vi "SetAdapTorrLocal_v0.vi"(2 "Debug Mode":bool, 3 "Elapsed Time (s)":dbl, 4 "State":enum16{"Edit", "Start", "Run", "End", "Idle"}(ring), 5 "Argument List In":string[](array[string])) -> (0 "Status Out":string, 1 "Argument List Out":string[](array[string]))   [LabVIEW 2011]
panel:
  in  "error in (no error)":errorcluster
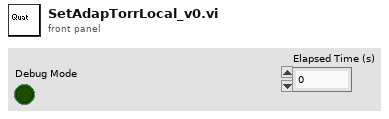
[diagram p1: front panel]
types:
  T1 = enum16{"Discrete", "Continuous", "Instantaneous"}
  T2 = enum32{"Invalid", "Default", "Floating", "Floating/Auto-Hide", "Modal"}
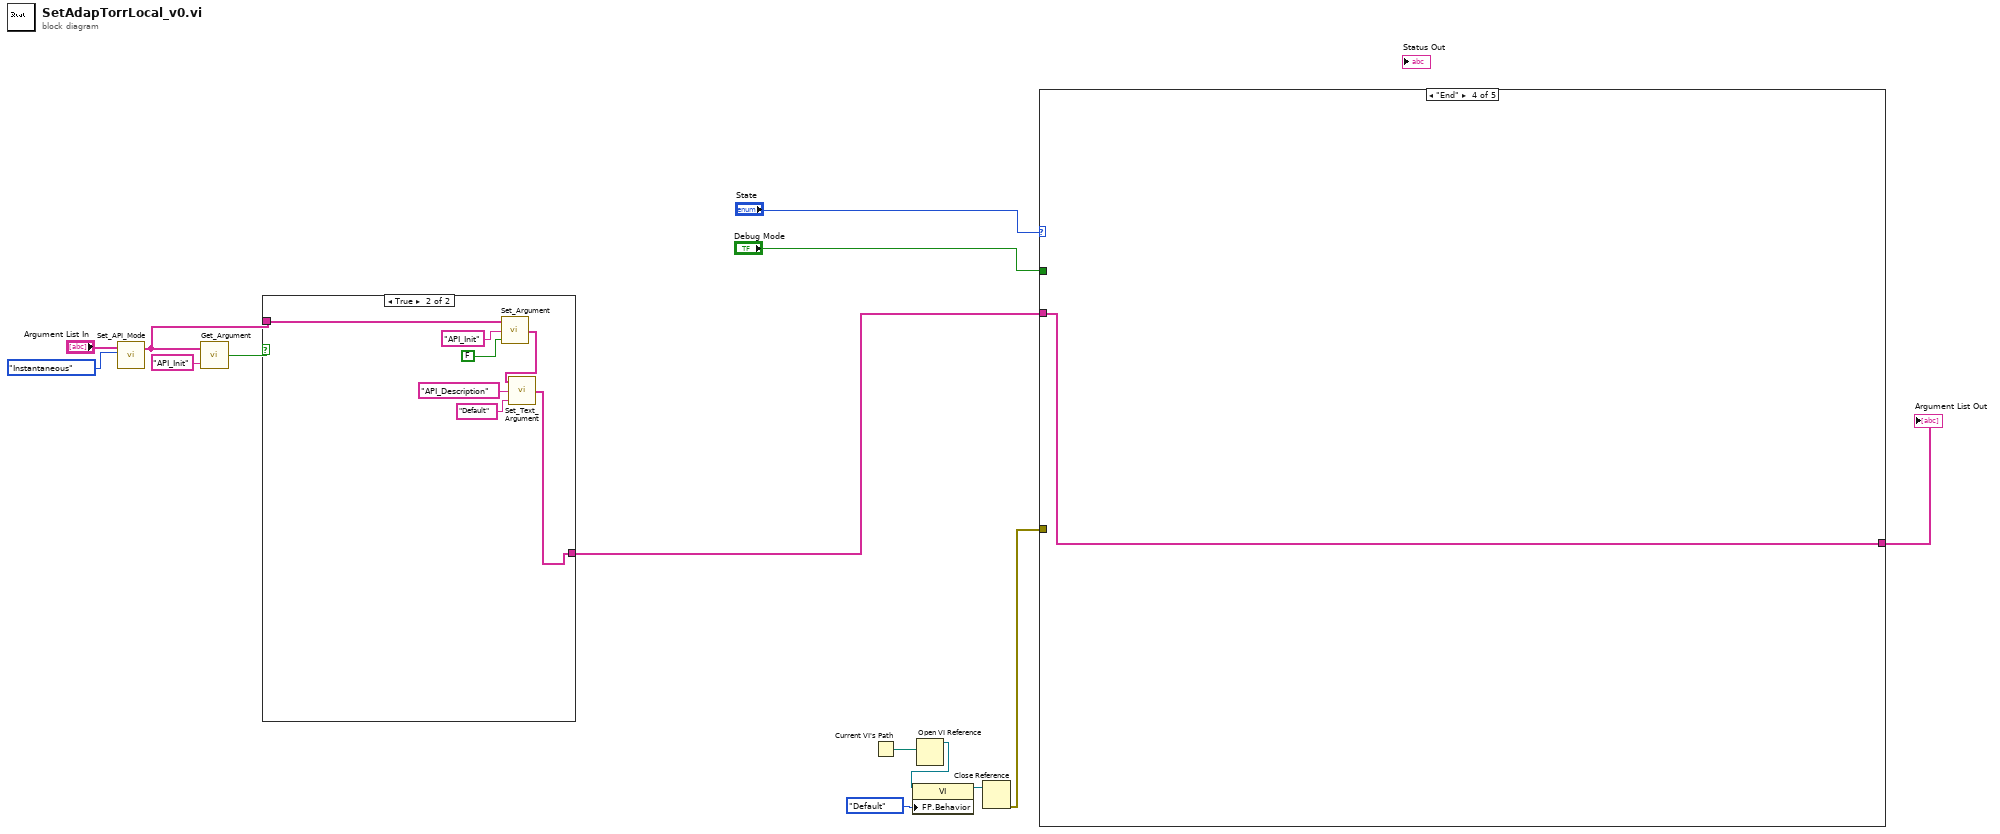
[diagram p0: block diagram]
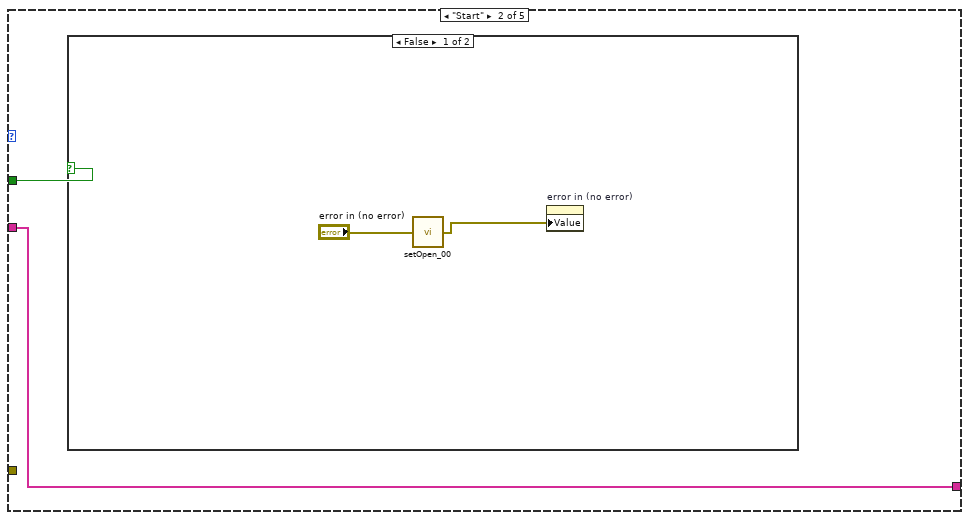
[diagram p4: hidden frame]
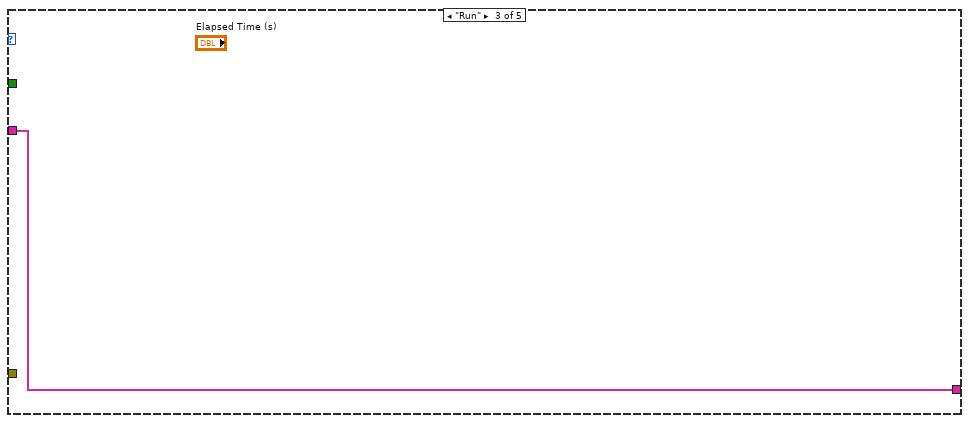
[diagram p6: hidden frame]
diagram:
  n1 = call "Set_API_Mode.vi"("API Mode"=T1."Instantaneous", "Argument List In"="Argument List In") -> ("Argument List Out"=w2:string[])  [unwired: 3 in]
  n2 = call "Get_Argument.vi"("Argument"="API_Init", "Argument List"=w2) -> ("Enabled"=w3:bool)
  n3 = case shown="True" w3 {
    tunnel: w2 -> [w15 w22]
    tunnel: [w15 w16] -> w1
    frame False {
    }
    frame True {
      n4 = call "Set_Argument.vi"("Enable"=FALSE, "Argument"="API_Init", "Argument List In"=w22) -> ("Argument List Out"=w19:string[])
      n5 = call "Set_Text_Argument.vi"("Text"="Default", "Argument"="API_Description", "Argument List In"=w19) -> ("Argument List Out"=w16:string[])
    }
  }
  n6 = Current VI's Path() -> (path=w11:path)
  n7 = Open VI Reference(vi path=w11) -> (vi reference=w10:refnum<vi>)  [unwired: 1 in, 5 out]
  n8 = property class="VI"(reference=w10, "FP.Behavior"=T2."Default" ("Front Panel Window:Behavior")) -> (reference out=w8:refnum<vi>)  [unwired: 1 in, 1 out]
  n9 = Close Reference(reference=w8) -> (error out=w7:errorcluster)  [unwired: 1 in]
  n10 = case shown="\"End\"" "State" {
    tunnel: [w23 w25 w28 w29 w30] -> w13
    tunnel: w1 -> [w23 w25 w28 w29 w30]
    tunnel: "Debug Mode" -> [_ w24 _ _ _]
    tunnel: w7 -> [_ _ _ _ _]
    frame "Edit", Default {
    }
    frame "Start" {
      n11 = case shown="False" w24 {
        frame False {
          n12 = call "setOpen_00.vi"("error in (no error)"="error in (no error)") -> ("error out"=w26:errorcluster)
          n13 = property on="error in (no error)" class="Clust (strict)"("Value"=w26) -> ()  [unwired: 2 in, 2 out]
        }
        frame True {
        }
      }
    }
    frame "Run" {
    }
    frame "End" {
    }
    frame "Idle" {
    }
  }
  "Argument List Out" <- w13
